vi "Update_PositionProfileMove.vi"(6 "Skip Update?":bool, 8 "error in (no error)":errorcluster, 9 "StatusWord":u16, 10 "ControlWord":u16 format="%.0b", 11 "SoftmotionAxis in":refnum<class "SoftmotionAxis.lvclass">) -> (0 "error out":errorcluster, 1 "StatusWord Out":u16, 3 "SoftmotionAxis out":refnum<class "SoftmotionAxis.lvclass">)   [LabVIEW 2017, in "SoftmotionAxis.lvclass"]
uses:
  SoftmotionAxis.lvclass
  Utilities/Bit Manipulation.lvlib
  <resource>/objmgr/nimcai.rc
  <resource>/objmgr/nimotion.rc
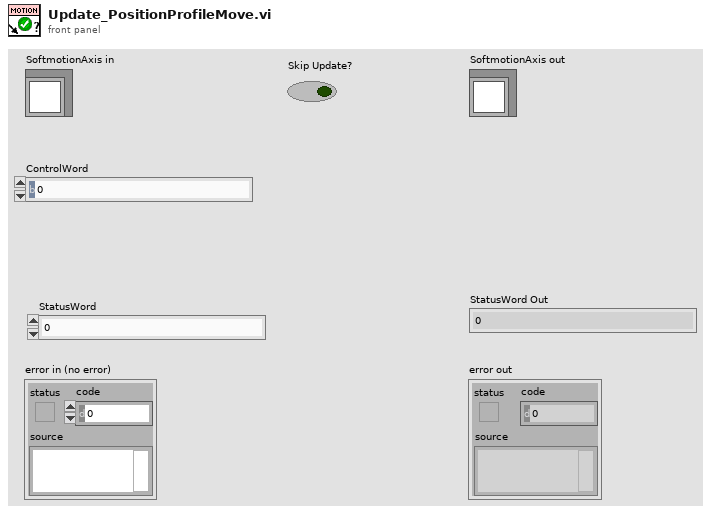
[diagram p1: front panel]
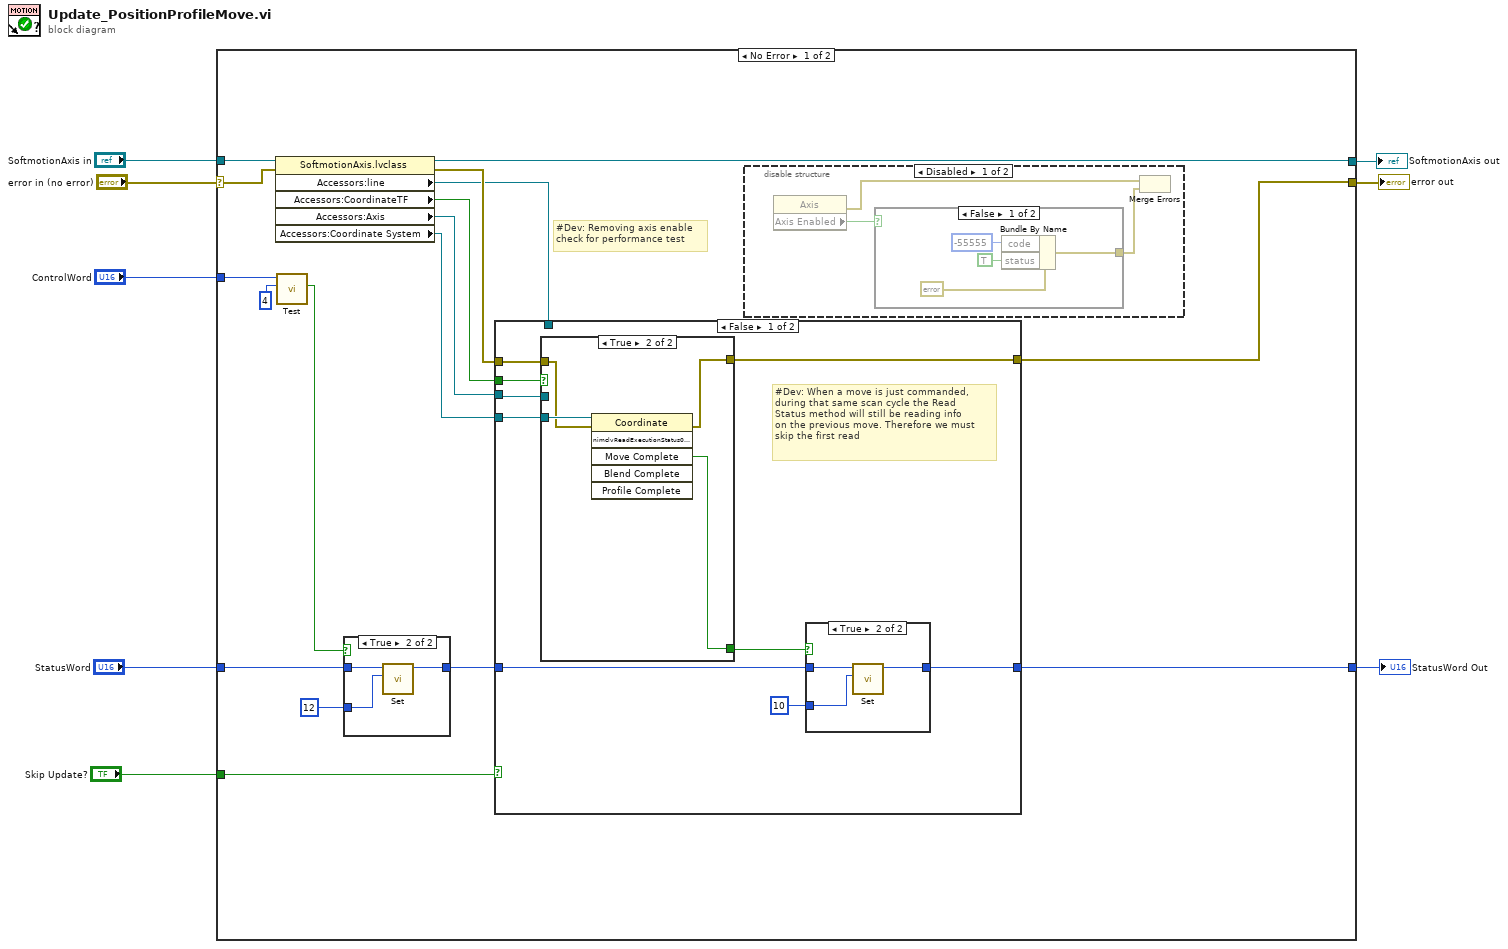
[diagram p0: block diagram]
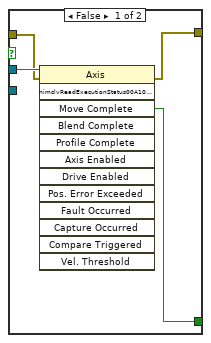
[diagram p4: hidden frame]
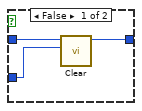
[diagram p5: hidden frame]
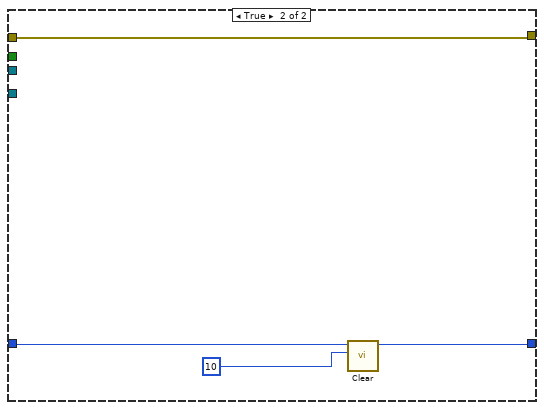
[diagram p6: hidden frame]
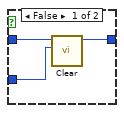
[diagram p7: hidden frame]
diagram:
  n1 = case shown="No Error" "error in (no error)" {
    selector: "error in (no error)" -> [w23 w68]
    tunnel: [w10 w68] -> w7
    tunnel: [w16 w67] -> w5
    tunnel: "SoftmotionAxis in" -> [w24 w67]
    tunnel: "StatusWord" -> [w22 w66]
    tunnel: [w25 w66] -> w3
    tunnel: "ControlWord" -> [w20 _]
    tunnel: "Skip Update?" -> [w15 _]
    frame No Error {
      # "#Dev: Removing axis enable\ncheck for performance test"
      n2 = property class="SoftmotionAxis.lvclass"(reference=w24, error in=w23) -> (reference out=w16:refnum<class "SoftmotionAxis.lvclass">, error out=w11:errorcluster, "Accessors:line"=w9:refnum<k20>, "Accessors:CoordinateTF"=w14:bool, "Accessors:Axis"=w13:refnum<k21>, "Accessors:Coordinate System"=w12:refnum<k21>)
      n3 = call "Test.vi"("Bit to test"=u8 4, "Data_In"=w20) -> ("bit value"=w18:bool)  [unwired: 8 in, 1 out]
      n4 = case shown="True" w18 {
        tunnel: w22 -> [w62 w64]
        tunnel: [w61 w65] -> w21
        tunnel: u8 12 -> [w60 w63]
        frame False {
          n5 = call "Clear.vi"("Bit to clear"=w60, "Data_In"=w62) -> ("Data_Out"=w61:u16)  [unwired: 9 in]
        }
        frame True {
          n6 = call "Set.vi"("Bit to set"=w63, "Data_In"=w64) -> ("Data_Out"=w65:u16)  [unwired: 9 in]
        }
      }
      n7 = case shown="False" w15 {
        tunnel: [w40 w59] -> w25
        tunnel: w21 -> [w39 w58]
        tunnel: w13 -> [w38 _]
        tunnel: w14 -> [w36 _]
        tunnel: w12 -> [w35 _]
        tunnel: w11 -> [w34 w56]
        tunnel: [w33 w56] -> w10
        tunnel: w9 -> [_ _]
        frame False {
          # "#Dev: When a move is just commanded, \nduring that same scan cycle the Read\nStatus method will still be reading info\non the previous move. Therefore we must\nskip the first read"
          n8 = case shown="True" w36 {
            tunnel: w38 -> [w45 _]
            tunnel: [w44 w48] -> w37
            tunnel: w35 -> [_ w49]
            tunnel: w34 -> [w43 w47]
            tunnel: [w42 w46] -> w33
            frame False {
              n9 = invoke class="Axis" method="nimclvReadExecutionStatus00A10001"(reference=w45, error in=w43) -> (error out=w42:errorcluster, "Move Complete"=w44:bool)  [unwired: 11 in, 11 out]
            }
            frame True {
              n10 = invoke class="Coordinate" method="nimclvReadExecutionStatus00A10011"(reference=w49, error in=w47) -> (error out=w46:errorcluster, "Move Complete"=w48:bool)  [unwired: 4 in, 4 out]
            }
          }
          n11 = case shown="True" w37 {
            tunnel: w39 -> [w52 w55]
            tunnel: [w51 w54] -> w40
            tunnel: u8 10 -> [w50 w53]
            frame False {
              n12 = call "Clear.vi"("Bit to clear"=w50, "Data_In"=w52) -> ("Data_Out"=w51:u16)  [unwired: 9 in]
            }
            frame True {
              n13 = call "Set.vi"("Bit to set"=w53, "Data_In"=w55) -> ("Data_Out"=w54:u16)  [unwired: 9 in]
            }
          }
        }
        frame True {
          n14 = call "Clear.vi"("Bit to clear"=u8 10, "Data_In"=w58) -> ("Data_Out"=w59:u16)  [unwired: 9 in]
        }
      }
      n15 = disable-structure shown="Disabled" {
        frame Disabled {
          n16 = property class="Axis"() -> (error out=w26:errorcluster, "Axis Enabled"=w28:bool)  [unwired: 2 in, 1 out]
          n17 = case shown="False" w28 {
            tunnel: [w29 _] -> w27
            frame False {
              n18 = Bundle By Name(cluster=errorcluster {"status"=FALSE, "code"=0, "source"=""} ("error in (no error)"), "code"=-55555, "status"=TRUE) -> (w29:errorcluster)
            }
            frame True {
            }
          }
          n19 = Merge Errors(w26, w27) -> ()  [unwired: 1 out]
        }
        frame Enabled {
        }
      }
    }
    frame Error {
    }
  }
  "error out" <- w7
  "SoftmotionAxis out" <- w5
  "StatusWord Out" <- w3
